vi "Read UID.vi"(11 "Teller in":refnum<class "Teller.lvclass">) -> (2 "UID":string)   [LabVIEW 2020, in "jettl.lvlib" / "Teller.lvclass"]
uses:
  Teller.lvclass
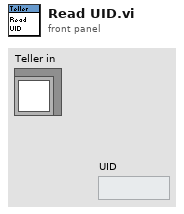
[diagram p1: front panel]
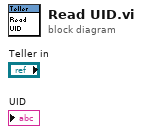
[diagram p0: block diagram]
diagram:
